vi "Simple Example.vi"() -> ()   [LabVIEW 2020]
uses:
  <vilib>/Instr/_visa.llb/VISA Configure Serial Port (Instr).vi
panel:
  out "Infusion rate(ul/s)":dbl
  out "Infused Volume (ul)":dbl
  out "Status":string
  in  "stop":bool
  out "read buffer":string
  out "error out":errorcluster
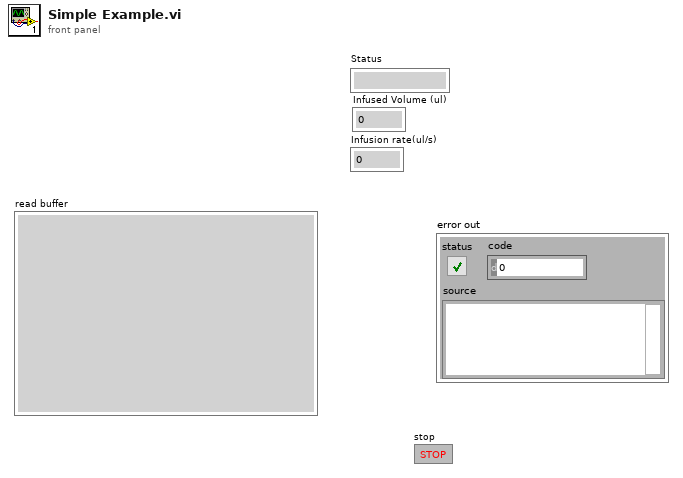
[diagram p1: front panel]
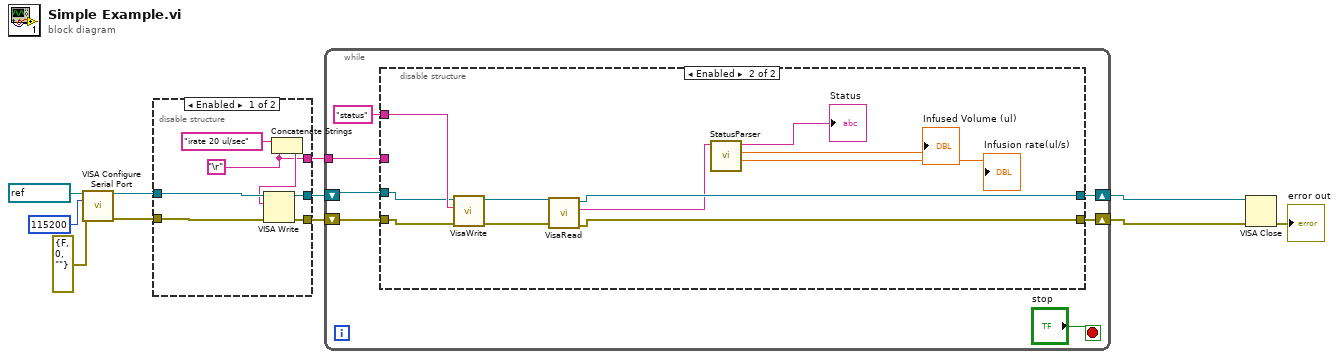
[diagram p0: block diagram]
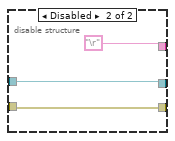
[diagram p2: hidden frame]
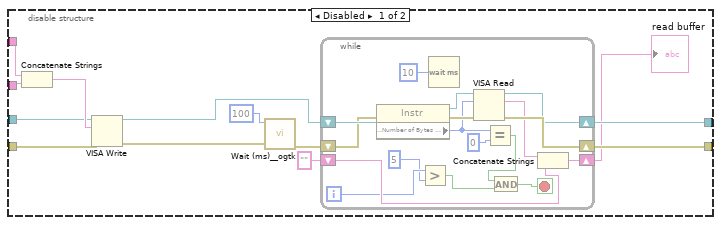
[diagram p3: hidden frame]
diagram:
  n1 = call-poly "VISA Configure Serial Port"("VISA resource name"=refnum<visa-resource-name> "COM4", "baud rate (9600)"=u32 115200, "error in (no error)"=errorcluster {"status"=FALSE, "code"=0, "source"=""}) -> ("VISA resource name out"=w5:refnum<visa-resource-name>, "error out"=w8:errorcluster)  [unwired: 11 in]
  n2 = disable-structure shown="Enabled" {
    disable-tunnel: w8 -> [w18 w19]
    disable-tunnel: w5 -> [w17 w20]
    disable-tunnel: [w16 w20] -> w4
    disable-tunnel: [w14 w19] -> w2
    disable-tunnel: [w13 "\r"] -> w1
    frame Enabled {
      w13 = "\r"
      n3 = Concatenate Strings("irate 20 ul/sec" ("string"), w13) -> (w15:string)
      n4 = VISA Write(VISA resource name=w17, write buffer=w15, error in (no error)=w18) -> (VISA resource name out=w16:refnum<visa-resource-name>, error out=w14:errorcluster)  [unwired: 1 out]
    }
    frame Disabled {
    }
  }
  n5 = while {
    tunnel: w1 -> [w24]
    shift-right: [w28] -> w11
    shift-left: w4 -> [w22]
    shift-right: [w27] -> w10
    shift-left: w2 -> [w26]
    stop <- "stop" stop-if-true
    n6 = disable-structure shown="Enabled" {
      disable-tunnel: [w41 w64] -> w28
      disable-tunnel: [w40 w63] -> w27
      disable-tunnel: w26 -> [w35 w69]
      disable-tunnel: "status" ("write buffer") -> [w33 w68]
      disable-tunnel: w24 -> [w32 _]
      disable-tunnel: w22 -> [w29 w67]
      frame Disabled {
        n7 = Concatenate Strings(w33, w32) -> (w31:string)
        n8 = VISA Write(VISA resource name=w29, write buffer=w31, error in (no error)=w35) -> (VISA resource name out=w30:refnum<visa-resource-name>, error out=w34:errorcluster)  [unwired: 1 out]
        n9 = call <userlib>:"Wait (ms)__ogtk.vi"("error in (no error)"=w34, "milliseconds to wait"=u32 100) -> ("error out"=w38:errorcluster)  [unwired: 8 in, 1 out]
        n10 = while {
          shift-right: [w57] -> w41
          shift-left: w30 -> [w56]
          shift-right: [w58] -> w40
          shift-left: w38 -> [w53]
          shift-right: [w52] -> w39
          shift-left: "" -> [w51]
          i -> [w43]
          stop <- w46 stop-if-true
          n11 = property class="Instr"(reference=w56, error in=w53) -> (reference out=w55:refnum<visa-resource-name>, error out=w54:errorcluster, "Serial Settings:Number of Bytes at Serial Port"=w49:u32)
          n12 = Greater?(x=w43, y=5 ("x")) -> (0:w44:bool)
          n13 = Wait (ms)(milliseconds to wait=u32 10) -> ()  [unwired: 1 out]
          n14 = VISA Read(VISA resource name=w55, byte count=w49, error in (no error)=w54) -> (VISA resource name out=w57:refnum<visa-resource-name>, read buffer=w50:string, error out=w58:errorcluster)  [unwired: 1 out]
          n15 = Equal?(x=w49, y=u32 0) -> (x = y?=w45:bool)
          n16 = And(x=w45, y=w44) -> (x .and. y?=w46:bool)
          n17 = Concatenate Strings(w50, w51) -> (w52:string)
        }
        "read buffer" <- w39
      }
      frame Enabled {
        n18 = call "VisaWrite.vi"("error in (no error)"=w69, "command"=w68, "VISA resource name"=w67) -> ("error out"=w66:errorcluster, "VISA resource name out"=w65:refnum<visa-resource-name>)  [unwired: 7 in]
        n19 = call "VisaRead.vi"("error out"=w66, "VISA resource name in"=w65) -> ("error out"=w63:errorcluster, "output"=w62:string, "VISA resource name out"=w64:refnum<visa-resource-name>)  [unwired: 7 in]
        n20 = call "StatusParser.vi"("Input String"=w62) -> ("Infusion rate(ul/s)"=→"Infusion rate(ul/s)":dbl, "Infused Volume (ul)"=→"Infused Volume (ul)":dbl, "Status"=→"Status":string)  [unwired: 8 in]
      }
    }
  }
  n21 = VISA Close(VISA resource name=w11, error in (no error)=w10) -> (error out=→"error out":errorcluster)
